vi "Get AI StringsAndValues.vi"(8 "error in (no error)":errorcluster, 11 "Instrument.Lockin in":refnum<class "Instrument.Lockin.lvclass">) -> (0 "error out":errorcluster, 2 "AI StringsAndValues":cluster{string, i32}[](array[cluster]), 3 "Instrument.Lockin out":refnum<class "Instrument.Lockin.lvclass">)   [LabVIEW 2019, in "Instrument.Lockin.lvclass"]
uses:
  Instrument.Lockin.lvclass
  Instrument.DAQ/Instrument.DAQ.lvclass
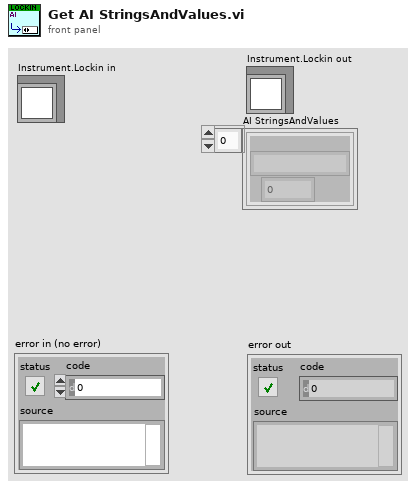
[diagram p1: front panel]
types:
  T1 = typedef "Instrument.DAQ.lvclass/DAQ.AI.Config--Config--Array.ctl" = T2[]
  T2 = typedef "Instrument.DAQ.lvclass/DAQ.AI.Config--Cluster.ctl" = cluster{"Channels":tag, "Coupling":T3, "Range":T4, "input terminal configuration":i32, "Type":T5}
  T3 = typedef "Instrument.DAQ.lvclass/DAQ.AI.Coupling--enum.ctl" = u16
  T4 = typedef "Instrument.DAQ.lvclass/DAQ.AI.Range--enum.ctl" = enum16{"±0.316", "±1.00", "±3.16", "±10.0", "±31.6", "±42.4"}
  T5 = typedef "Instrument.DAQ.lvclass/DAQ.Type--enum.ctl" = enum16{"None", "USB 4431", "PXI 446x"}
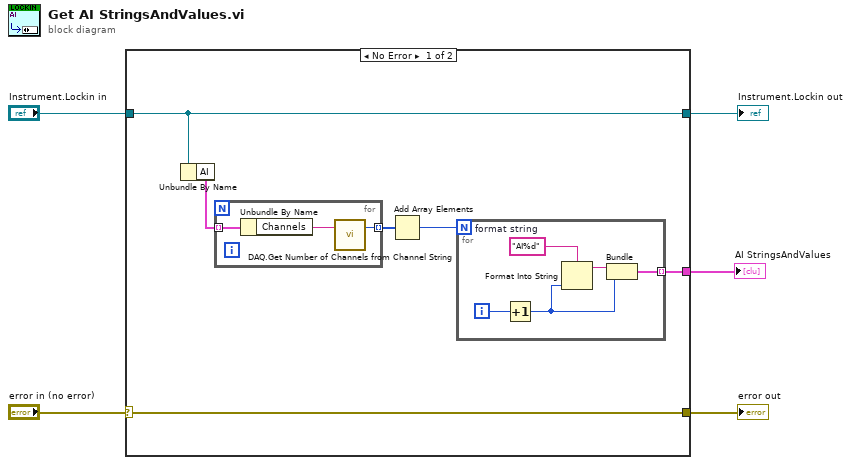
[diagram p0: block diagram]
diagram:
  n1 = case shown="No Error" "error in (no error)" {
    selector: "error in (no error)" -> [w8 w20]
    tunnel: "Instrument.Lockin in" -> [w9 w21]
    tunnel: [w9 w21] -> w4
    tunnel: [w8 w20] -> w2
    tunnel: [w6 _] -> w1
    frame No Error {
      n2 = Unbundle By Name(w9) -> ("AI"=w11:T1)
      n3 = for {
        tunnel: w11 -> [w14] mode=indexing
        tunnel: [w13] -> w10 mode=indexing
        n4 = Unbundle By Name(w14) -> ("Channels"=w12:tag)
        n5 = call "DAQ.Get Number of Channels from Channel String.vi"("Channels String"=w12) -> ("# channels"=w13:i32)  [unwired: 2 in]
      }
      n6 = Add Array Elements(numeric array=w10) -> (sum=w7:i32)
      n7 = for {
        N: w7 -> [_]
        tunnel: [w19] -> w6 mode=indexing
        i -> [w17]
        w18 = "AI%d"  # format string
        n8 = Increment(x=w17) -> (x+1=w16:i32)
        n9 = Format Into String(format string=w18, w16) -> (resulting string=w15:string)  [unwired: 2 in, 1 out]
        n10 = Bundle(w15, w16) -> (w19:cluster{string, i32})  [unwired: 1 in]
      }
    }
    frame Error {
    }
  }
  "Instrument.Lockin out" <- w4
  "error out" <- w2
  "AI StringsAndValues" <- w1
